vi "FGV_HovaCAL_Interface_Kommunikation.vi"(8 "error in":errorcluster, 9 "Logging":bool, 10 "Stop":bool, 11 "Aktion":T1) -> (0 "error out":errorcluster, 2 "connected?":bool, 3 "Aktion out":T1)   [LabVIEW 2020, in "Linearisierung v2.lvlib" / "Gasteiler.lvlib" / "HovaCAL_Interface.lvlib" / "Kommunikation.lvlib"]
uses:
  Kommunikation.lvlib
  Aktion_FGV_HovaCAL_Interface_Kommunikation.ctl
  Aktion_FGV_HovaCAL_Interface_GetData.ctl
  Aktion_FGV_HovaCAL_Interface_SetData.ctl
  Aktion_FGV_HovaCAL_Interface_Gasliste.ctl
  Aktionen FGV Gasteiler Daten.ctl
  KGN/KGN.lvlib
  Gasteiler.lvlib
  KGN/set/set.lvlib
  KGN/GUI Get/KGN GUI Get.lvlib
  KGN/GUI Set/KGN GUI Set.lvlib
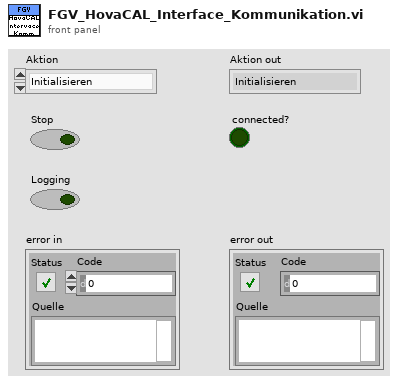
[diagram p1: front panel]
types:
  T1 = typedef "Linearisierung v2.lvlib/Gasteiler.lvlib/HovaCAL_Interface.lvlib/Kommunikation.lvlib/Aktion_FGV_HovaCAL_Interface_Kommunikation.ctl" = enum16{"Initialisieren", "Set Konzentrationen", "Set Gase", "Set Limits", "Get Dynamische Werte", "Beenden", "Com ändern", "Get Gase init", "Pause", "Get Gasteiler Infos", "Get MFC Infos", "Set Pumpen Parameter", "Set Pumpe Konzenration", "Set Pumpe run", "Set Temperaturen", "Set Fluss", "Get Gase", "Get Limits", "Get Dynamische Werte 1", "Get Dynamische Werte 2"}
  T2 = cluster{"first contact in":bool, "first actual values in ":bool}
  T3 = typedef "Linearisierung v2.lvlib/Gasteiler.lvlib/HovaCAL_Interface.lvlib/Kommunikation.lvlib/Aktion_FGV_HovaCAL_Interface_GetData.ctl" = enum16{"lesen", "SystemInfo", "MFC Info", "actual Values", "Limits", "first contact"}
  T4 = cluster{"Serial Settings:Baud Rate":u32, "Serial Settings:Data Bits":u16, "Serial Settings:Parity":u16, "Serial Settings:Stop Bits":u16, "Serial Settings:Flow Control":u16, "Enable Termination Char (T)":bool, "Message Based Settings:Termination Character":u8}
  T5 = typedef "Linearisierung v2.lvlib/Gasteiler.lvlib/HovaCAL_Interface.lvlib/Kommunikation.lvlib/Aktion_FGV_HovaCAL_Interface_SetData.ctl" = enum16{"lesen", "Konzentrationen", "Pumpen Parameter", "Pumpe Konzentration", "Pumpe run", "Temperaturen", "Fluss", "Limits", "init"}
  T6 = typedef "Linearisierung v2.lvlib/Gasteiler.lvlib/HovaCAL_Interface.lvlib/Kommunikation.lvlib/Aktion_FGV_HovaCAL_Interface_Gasliste.ctl" = enum16{"lesen", "setzen", "erstellen"}
  T7 = typedef "Linearisierung v2.lvlib/Gasteiler.lvlib/Aktionen FGV Gasteiler Daten.ctl" = enum16{"lesen", "Gasteiler Daten", "Seriellen Param.", "MB-Endwert", "laden", "speichern", "Anforderung", "TCP", "Aufzeichnung Start"}
  T8 = cluster{"input concentration setpoint":dbl, "output concentration setpoint":dbl}[]
  T9 = typedef "Linearisierung v2.lvlib/Gasteiler.lvlib/HovaCAL_Interface.lvlib/Controls.lvlib/Info Cluster.ctl" = cluster{"device":string, "version":string, "number of mfc":i32, "number of pumps":i32, "number of temp controllers":i32, "number of mfs":i32, "number of balances":i32}
  T10 = typedef "Linearisierung v2.lvlib/Gasteiler.lvlib/HovaCAL_Interface.lvlib/Controls.lvlib/Pump Concentration Mode.ctl" = i32
  T11 = typedef "Linearisierung v2.lvlib/Gasteiler.lvlib/HovaCAL_Interface.lvlib/Controls.lvlib/Reagent.ctl" = i32
  T12 = cluster{"concentratio mode":T10, "Reagent":T11, "Molarity":dbl, "density":dbl, "syringe":dbl, "pump_a":dbl}[]
  T13 = typedef "Linearisierung v2.lvlib/Gasteiler.lvlib/HovaCAL_Interface.lvlib/Controls.lvlib/Pump Concentration.ctl" = cluster{"reagent conc SP":dbl, "water conc SP":dbl}
  T14 = typedef "Linearisierung v2.lvlib/Gasteiler.lvlib/HovaCAL_Interface.lvlib/Controls.lvlib/Pump Dry Mode.ctl" = i32
  T15 = typedef "Linearisierung v2.lvlib/Gasteiler.lvlib/HovaCAL_Interface.lvlib/Controls.lvlib/Pump Control Mode.ctl" = u32
  T16 = cluster{"running?":bool, "dry mode":T14, "control mode":T15}
  T17 = cluster{"Input Concentrations (Ausgang)":cluster{"input concentration setpoint":dbl, "output concentration setpoint":dbl, "output concentration":dbl, "output concentration dry":dbl}[], "Cluster":cluster{"Temp Cluster":cluster{"temp SP":dbl, "temp":dbl, "humidity":dbl}[], "PumpModeGeneral-Cluster":cluster{"running?":bool, "dry mode":T14, "control mode":T15}, "PumpMode-Cluster":cluster{"Speed":dbl, "concentratio mode":T10, "Reagent":T11, "Molarity":dbl, "density":dbl, "syringe":dbl, "pumpe_a":dbl}[], "Pump Concentrations-Cluster":cluster{"reagent conc SP":dbl, "reagent conc":dbl, "reagent conc dry":dbl, "water conc SP":dbl, "water conc":dbl, "water conc dry":dbl}[], "Flow Output Cluster (Ausgang)":cluster{"total flow setpoint":dbl, "total flow":dbl}, "Pump MassFlow-Cluster":cluster{"reagent mf SP":dbl, "reagent mf":dbl, "water mf SP":dbl, "water mf":dbl, "water/reagent mf SP":dbl, "water/reagent mf":dbl}[], "MFC Flows-Cluster":cluster{"MFC  actual flow l/min":dbl, "MFC expected flow l/min":dbl}[]}}
  T18 = cluster{"Input Concentrations (Ausgang)":cluster{"input concentration setpoint":dbl, "output concentration setpoint":dbl, "output concentration":dbl, "output concentration dry":dbl}[], "Cluster":cluster{"Temp Cluster":cluster{"temp SP":dbl, "temp":dbl, "humidity":dbl}[], "PumpModeGeneral-Cluster":cluster{"running?":bool, "dry mode":T14, "control mode":T15}, "Flow Output Cluster (Ausgang)":cluster{"total flow setpoint":dbl, "total flow":dbl}, "MFC Flows (Ausgang)":cluster{"MFC  actual flow l/min":dbl, "MFC expected flow l/min":dbl}[]}}
  T19 = cluster{"input concentration setpoint":dbl, "output concentration setpoint":dbl, "output concentration":dbl, "output concentration dry":dbl}[]
  T20 = cluster{"temp SP":dbl, "temp":dbl, "humidity":dbl}[]
  T21 = cluster{"total flow setpoint":dbl, "total flow":dbl}
  T22 = cluster{"MFC  actual flow l/min":dbl, "MFC expected flow l/min":dbl}[]
  T23 = cluster{"Cluster":cluster{"PumpMode-Cluster":cluster{"Speed":dbl, "concentratio mode":T10, "Reagent":T11, "Molarity":dbl, "density":dbl, "syringe":dbl, "pumpe_a":dbl}[], "Pump Concentrations-Cluster":cluster{"reagent conc SP":dbl, "reagent conc":dbl, "reagent conc dry":dbl, "water conc SP":dbl, "water conc":dbl, "water conc dry":dbl}[], "Pump MassFlow-Cluster":cluster{"reagent mf SP":dbl, "reagent mf":dbl, "water mf SP":dbl, "water mf":dbl, "water/reagent mf SP":dbl, "water/reagent mf":dbl}[]}}
  T24 = cluster{"Speed":dbl, "concentratio mode":T10, "Reagent":T11, "Molarity":dbl, "density":dbl, "syringe":dbl, "pumpe_a":dbl}[]
  T25 = cluster{"reagent conc SP":dbl, "reagent conc":dbl, "reagent conc dry":dbl, "water conc SP":dbl, "water conc":dbl, "water conc dry":dbl}[]
  T26 = cluster{"reagent mf SP":dbl, "reagent mf":dbl, "water mf SP":dbl, "water mf":dbl, "water/reagent mf SP":dbl, "water/reagent mf":dbl}[]
  T27 = typedef "AK-Schnittstelle.lvlib/AK Seriell.lvlib/Serielle Parameter.ctl" = cluster{"VISA resource name":refnum<visa-resource-name>, "baud rate":u32, "data bits":u16, "parity":u16, "stop bits":u16, "flow control":u16}
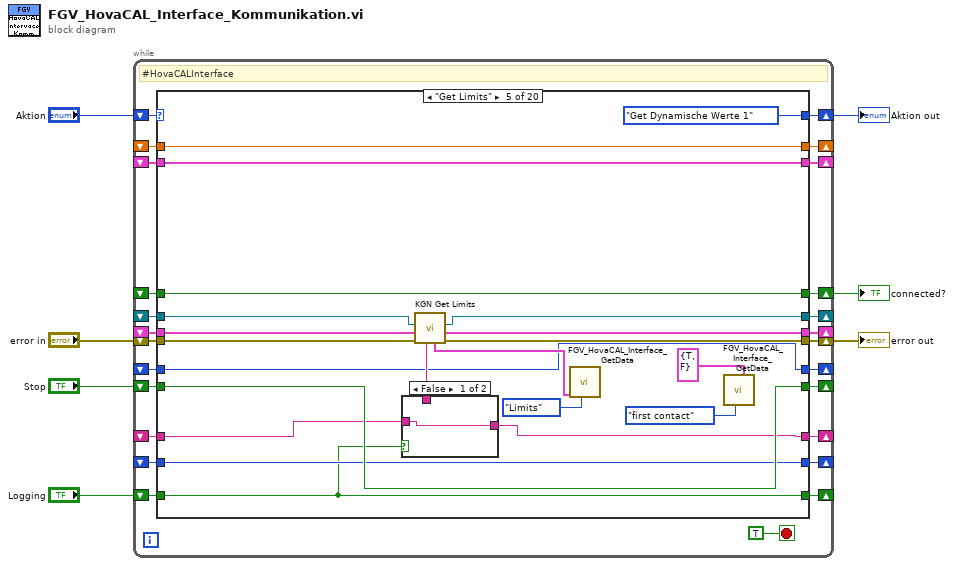
[diagram p0: block diagram]
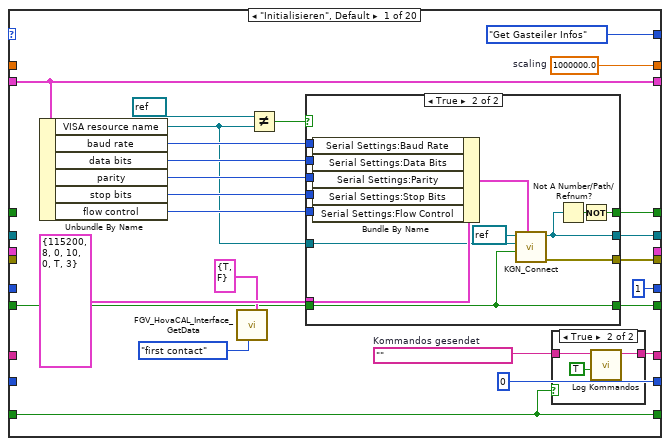
[diagram p2: hidden frame]
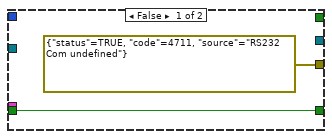
[diagram p4: hidden frame]
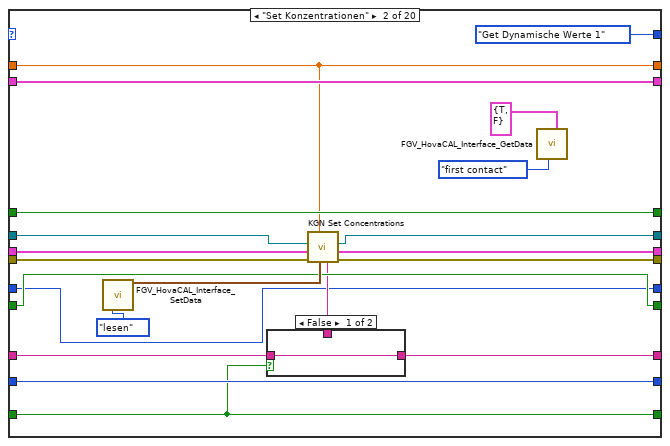
[diagram p5: hidden frame]
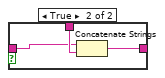
[diagram p6: hidden frame]
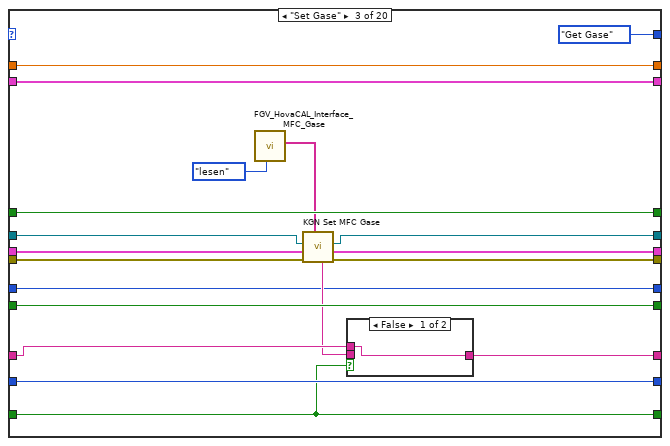
[diagram p7: hidden frame]
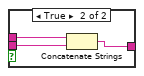
[diagram p8: hidden frame]
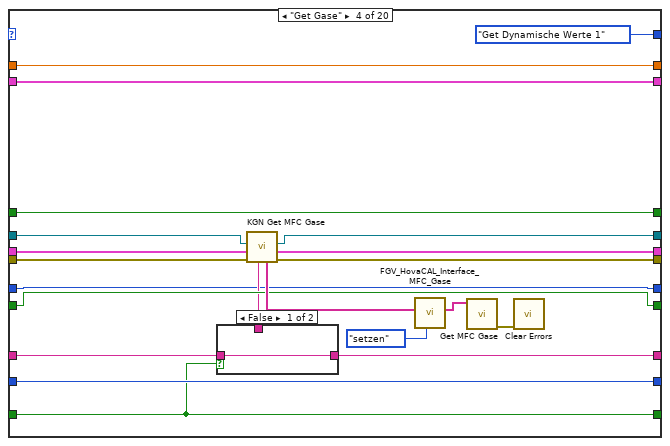
[diagram p9: hidden frame]
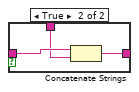
[diagram p10: hidden frame]
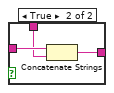
[diagram p11: hidden frame]
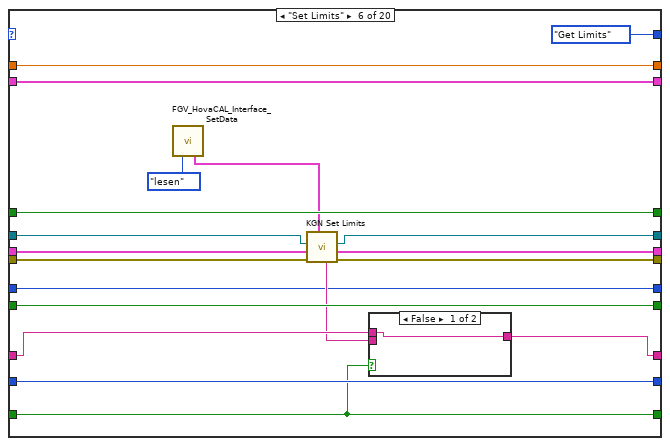
[diagram p12: hidden frame]
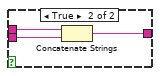
[diagram p13: hidden frame]
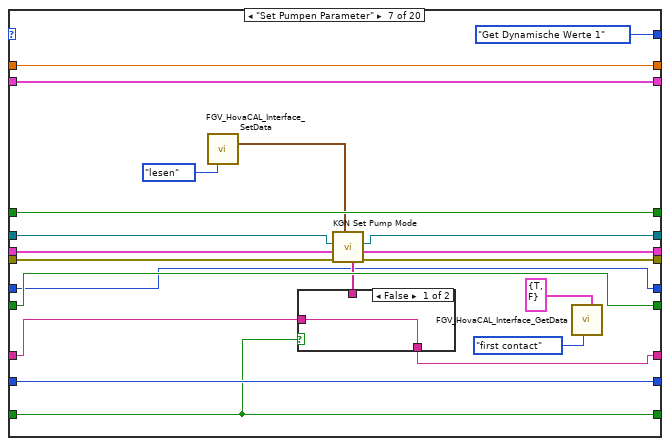
[diagram p14: hidden frame]
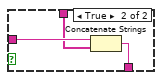
[diagram p15: hidden frame]
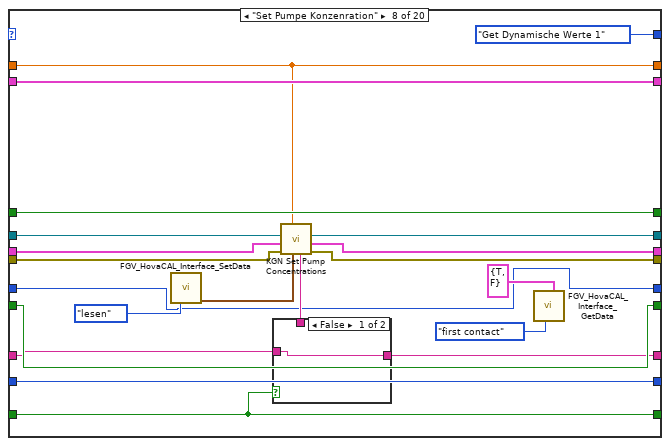
[diagram p16: hidden frame]
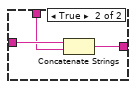
[diagram p17: hidden frame]
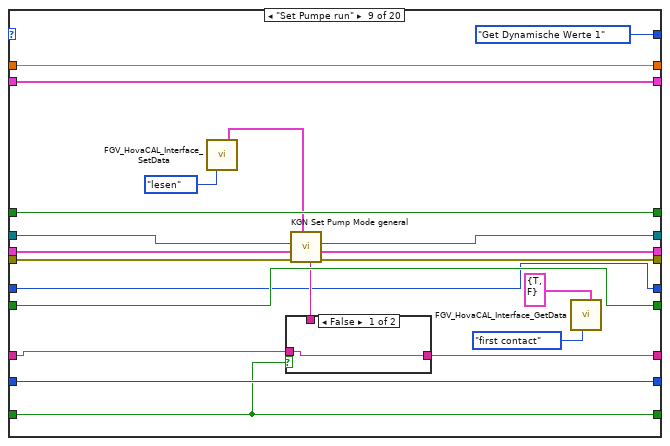
[diagram p18: hidden frame]
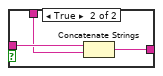
[diagram p19: hidden frame]
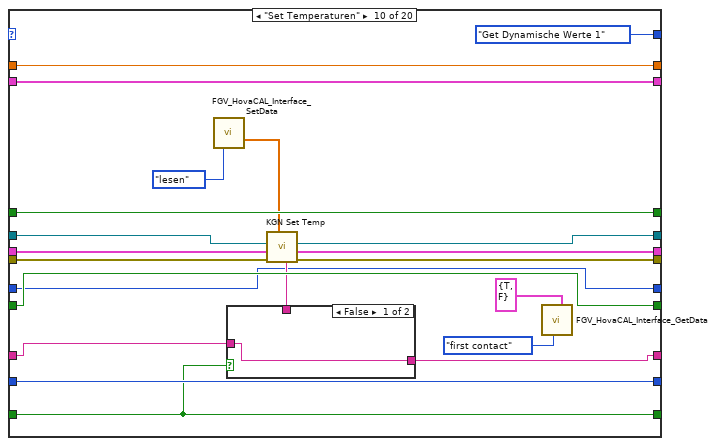
[diagram p20: hidden frame]
diagram:
  n1 = while {
    shift-right: [w29] -> w6
    shift-left: "error in" -> [w26]
    shift-right: [w31] -> _
    shift-left: _ -> [w30]
    shift-right: [w28] -> _
    shift-left: _ -> [w27]
    shift-right: [w25] -> w5
    shift-left: "Aktion" -> [w8]
    shift-right: [w24] -> _
    shift-left: _ -> [w23]
    shift-right: [w22] -> w4
    shift-left: _ -> [w21]
    shift-right: [w20] -> _
    shift-left: _ -> [w19]
    shift-right: [w17] -> _
    shift-left: "Stop" -> [w18]
    shift-right: [w16] -> _
    shift-left: _ -> [w15]
    shift-right: [w14] -> _
    shift-left: _ -> [w13]
    shift-right: [w11] -> _
    shift-left: "Logging" -> [w12]
    shift-right: [w10] -> _
    shift-left: _ -> [w9]
    stop <- TRUE stop-if-true
    # "#HovaCALInterface"
    n2 = case shown="\"Get Limits\"" w8 {
      selector: w8 -> [_ _ _ _ _ _ _ _ _ _ _ w334 w352 _ _ _ _ _ _ _]
      tunnel: [w56 w97 w120 w145 w170 w193 w218 w243 w268 w293 w317 w344 w380 w420 w453 w482 w492 w522 w548 w577] -> w31
      tunnel: w30 -> [w56 w97 w120 w145 w170 w193 w218 w243 w268 w293 w317 w344 w380 w420 w453 w482 w491 w522 w548 w577]
      tunnel: [w49 w90 w111 w136 w162 w184 w211 w236 w255 w287 w309 w340 w376 w416 w451 w479 w495 w514 w543 w563] -> w29
      tunnel: [w45 w94 w115 w140 w165 w188 w214 w238 w264 w285 w311 w342 w378 w418 w450 w481 w496 w517 w544 w565] -> w28
      tunnel: w27 -> [_ w95 w116 w141 w166 w189 w215 w241 w265 w289 w312 w343 w379 w419 w445 w481 w496 w518 w546 w575]
      tunnel: w26 -> [_ w91 w113 w138 w155 w187 w210 w237 w261 w288 w310 w341 w377 w417 w452 w479 w495 w513 w545 w574]
      tunnel: [Aktion_FGV_HovaCAL_Interface_Kommunikation."Get Gasteiler Infos" ("Aktion") Aktion_FGV_HovaCAL_Interface_Kommunikation."Get Dynamische Werte 1" ("Aktion") Aktion_FGV_HovaCAL_Interface_Kommunikation."Get Gase" ("Aktion") Aktion_FGV_HovaCAL_Interface_Kommunikation."Get Dynamische Werte 1" ("Aktion") Aktion_FGV_HovaCAL_Interface_Kommunikation."Get Dynamische Werte 1" ("Aktion") Aktion_FGV_HovaCAL_Interface_Kommunikation."Get Limits" ("Aktion") Aktion_FGV_HovaCAL_Interface_Kommunikation."Get Dynamische Werte 1" ("Aktion") Aktion_FGV_HovaCAL_Interface_Kommunikation."Get Dynamische Werte 1" ("Aktion") Aktion_FGV_HovaCAL_Interface_Kommunikation."Get Dynamische Werte 1" ("Aktion") Aktion_FGV_HovaCAL_Interface_Kommunikation."Get Dynamische Werte 1" ("Aktion") Aktion_FGV_HovaCAL_Interface_Kommunikation."Get Dynamische Werte 1" ("Aktion") w334 w351 Aktion_FGV_HovaCAL_Interface_Kommunikation."Get Dynamische Werte 1" ("Aktion") Aktion_FGV_HovaCAL_Interface_Kommunikation."Pause" ("Aktion") Aktion_FGV_HovaCAL_Interface_Kommunikation."Initialisieren" ("Aktion") w488 Aktion_FGV_HovaCAL_Interface_Kommunikation."Get Gase" ("Aktion") Aktion_FGV_HovaCAL_Interface_Kommunikation."Get MFC Infos" ("Aktion") Aktion_FGV_HovaCAL_Interface_Kommunikation."Get Gase init" ("Aktion")] -> w25
      tunnel: [_ w92 w112 w137 w163 w185 w212 w240 w262 w286 w316 w338 w374 w414 w448 w478 w494 w515 w540 w561] -> w24
      tunnel: w23 -> [_ w93 w114 w139 w164 w186 w213 w239 w263 w290 w316 w339 w375 w415 w448 w478 w494 w516 _ w572]
      tunnel: [w43 w96 w119 w144 w169 w192 w217 w242 w267 w292 w315 w335 w372 w412 w444 w477 w489 w520 w542 w573] -> w22
      tunnel: w21 -> [_ w96 w119 w144 w169 w192 w217 w242 w267 w292 w315 _ _ _ _ w477 w489 w520 w542 w573]
      tunnel: [w42 w89 w118 w143 w168 w191 w216 w235 w266 w291 w314 w333 w371 w411 w447 w476 w493 w519 w539 w569] -> w20
      tunnel: w19 -> [_ w89 w118 w143 w168 w191 w216 w235 w266 w291 w314 w333 w371 w411 w447 w476 w493 w519 w539 w569]
      tunnel: w18 -> [w39 w83 w108 w131 w157 w181 w204 w229 w254 w279 w304 w330 w359 w400 w441 w475 w487 w509 w535 w560]
      tunnel: [w38 w83 w108 w131 w157 w181 w204 w229 w254 w279 w304 w330 w359 w400 w441 w475 w487 w509 w535 w560] -> w17
      tunnel: [w35 w80 w105 w128 w154 w178 w202 w226 w251 w277 w301 w327 w356 w396 w437 w474 w486 w506 w531 w556] -> w16
      tunnel: w15 -> [_ w81 w107 w130 w156 w180 w203 w228 w253 w278 w303 w329 w357 w399 w440 w474 w486 w508 w530 w559]
      tunnel: [u32 0 w79 w104 w127 w152 w177 w200 w225 w250 w275 w300 w326 w354 w395 w438 w473 w485 w505 w529 w555] -> w14
      tunnel: w13 -> [_ w79 w104 w127 w152 w177 w200 w225 w250 w275 w300 w326 w354 w397 w438 w473 w485 w505 w529 w555]
      tunnel: w12 -> [w34 w78 w103 w126 w151 w176 w199 w224 w249 w274 w299 w325 w353 w394 w436 w472 w484 w504 w528 w554]
      tunnel: [w34 w78 w103 w126 w151 w176 w199 w224 w249 w274 w299 w325 w353 w394 w436 w472 w484 w504 w528 w554] -> w11
      tunnel: [u8 1 ("iteration out") w77 w102 w125 w150 w175 w198 w223 w248 w273 w298 w323 w349 w393 w435 w471 w483 w503 w527 w553] -> w10
      tunnel: w9 -> [_ w77 w102 w125 w150 w175 w198 w223 w248 w273 w298 w324 w350 w392 w435 w471 w483 w503 w527 w553]
      frame "Initialisieren", Default {
        w36 = ""  # Kommandos gesendet
        w42 = 1000000.0  # scaling
        n3 = Unbundle By Name(w56) -> ("VISA resource name"=w46:refnum<visa-resource-name>, "baud rate"=w54:u32, "data bits"=w53:u16, "parity"=w52:u16, "stop bits"=w51:u16, "flow control"=w50:u16)
        n4 = call "FGV_HovaCAL_Interface_GetData.vi"("first flags in"=T2 {"first contact in"=TRUE, "first actual values in "=FALSE}, "Aktion"=Aktion_FGV_HovaCAL_Interface_GetData."first contact") -> ()  [unwired: 5 in, 5 out]
        n5 = Not Equal?(x=refnum<visa-resource-name> refnum ("VISA-Ressourcenname"), y=w46) -> (x != y?=w47:bool)
        n6 = case shown="True" w47 {
          tunnel: T4 {"Serial Settings:Baud Rate"=115200, "Serial Settings:Data Bits"=8, "Serial Settings:Parity"=0, "Serial Settings:Stop Bits"=10, "Serial Settings:Flow Control"=0, "Enable Termination Char (T)"=TRUE, "Message Based Settings:Termination Character"=3} ("Serial Params in") -> [_ w76]
          tunnel: w54 -> [_ w74]
          tunnel: w53 -> [_ w73]
          tunnel: w52 -> [_ w72]
          tunnel: w51 -> [_ w71]
          tunnel: w50 -> [_ w70]
          tunnel: [errorcluster {"status"=TRUE, "code"=4711, "source"="RS232 Com undefined"} ("Fehler (Ausgang)") w69] -> w49
          tunnel: w46 -> [_ w68]
          tunnel: [_ w65] -> w45
          tunnel: [_ w64] -> w43
          tunnel: w39 -> [w61 w63]
          tunnel: [w61 w63] -> w38
          frame False {
          }
          frame True {
            n7 = Bundle By Name(cluster=w76, "Serial Settings:Baud Rate"=w74, "Serial Settings:Data Bits"=w73, "Serial Settings:Parity"=w72, "Serial Settings:Stop Bits"=w71, "Serial Settings:Flow Control"=w70) -> (w75:T4)
            n8 = call "KGN_Connect.vi"("Serial Params in"=w75, "Stopp"=w63, "serial port name"=w68, "VISA-Ressourcenname"=refnum<visa-resource-name> refnum) -> ("Fehler (Ausgang)"=w69:errorcluster, "VISA-Ressourcenname (Ausgang)"=w65:refnum<visa-resource-name>)  [unwired: 4 in, 2 out]
            n9 = Not A Number/Path/Refnum?(number/path/refnum=w65) -> (NaN/Path/Refnum?=w66:bool)
            n10 = Not(x=w66) -> (.not. x?=w64:bool)
          }
        }
        n11 = case shown="True" w34 {
          tunnel: w36 -> [w57 w60]
          tunnel: [w57 w59] -> w35
          frame False {
          }
          frame True {
            n12 = call "Log Kommandos.vi"("Init"=TRUE, "Kommandos"=w60) -> ("Kommandos out"=w59:string)  [unwired: 9 in]
          }
        }
      }
      frame "Set Konzentrationen" {
        n13 = call "FGV_HovaCAL_Interface_SetData.vi"("Aktion"=Aktion_FGV_HovaCAL_Interface_SetData."lesen") -> ("Set Values Cluster out"=w86:T8)  [unwired: 8 in, 6 out]
        n14 = call "KGN Set Concentrations.vi"("Set Values Cluster"=w86, "scaling"=w89, "Fehler (Eingang, kein Fehler)"=w91, "Info Cluster"=w93, "VISA-Referenz (Eingang)"=w95) -> ("Fehler (Ausgang)"=w90:errorcluster, "Info Cluster out"=w92:T9, "VISA-Referenz (Ausgang)"=w94:refnum<visa-resource-name>, "Kommandos gesendet"=w82:string)  [unwired: 2 in, 1 out]
        n15 = case shown="False" w78 {
          tunnel: w82 -> [_ w101]
          tunnel: w81 -> [w98 w100]
          tunnel: [w98 w99] -> w80
          frame False {
          }
          frame True {
            n16 = Concatenate Strings(w100, w101) -> (w99:string)
          }
        }
        n17 = call "FGV_HovaCAL_Interface_GetData.vi"("first flags in"=T2 {"first contact in"=TRUE, "first actual values in "=FALSE}, "Aktion"=Aktion_FGV_HovaCAL_Interface_GetData."first contact") -> ()  [unwired: 5 in, 5 out]
      }
      frame "Set Gase" {
        n18 = call "FGV_HovaCAL_Interface_MFC_Gase.vi"("Aktion"=Aktion_FGV_HovaCAL_Interface_Gasliste."lesen") -> ("mfc Gasnamen out"=w109:string[])  [unwired: 8 in, 2 out]
        n19 = call "KGN Set MFC Gase.vi"("mfc Gasnamen in"=w109, "Fehler (Eingang, kein Fehler)"=w113, "Info Cluster"=w114, "VISA-Referenz (Eingang)"=w116) -> ("Fehler (Ausgang)"=w111:errorcluster, "Info Cluster out"=w112:T9, "VISA-Referenz (Ausgang)"=w115:refnum<visa-resource-name>, "Kommandos gesendet"=w106:string)  [unwired: 3 in, 1 out]
        n20 = case shown="False" w103 {
          tunnel: w107 -> [w121 w124]
          tunnel: w106 -> [_ w123]
          tunnel: [w121 w122] -> w105
          frame False {
          }
          frame True {
            n21 = Concatenate Strings(w124, w123) -> (w122:string)
          }
        }
      }
      frame "Get Gase" {
        n22 = call "KGN Get MFC Gase.vi"("Fehler (Eingang, kein Fehler)"=w138, "Info Cluster"=w139, "VISA-Ressourcenname"=w141) -> ("Fehler (Ausgang)"=w136:errorcluster, "Info Cluster out"=w137:T9, "VISA-Ressourcenname out"=w140:refnum<visa-resource-name>, "mfc Gas"=w134:string[], "Kommandos gesendet"=w129:string)  [unwired: 3 in, 1 out]
        n23 = case shown="False" w126 {
          tunnel: w130 -> [w146 w149]
          tunnel: w129 -> [_ w148]
          tunnel: [w146 w147] -> w128
          frame False {
          }
          frame True {
            n24 = Concatenate Strings(w149, w148) -> (w147:string)
          }
        }
        n25 = call "FGV_HovaCAL_Interface_MFC_Gase.vi"("Aktion"=Aktion_FGV_HovaCAL_Interface_Gasliste."setzen", "mfc Gasnamen in"=w134) -> ("mfc Gasnamen out"=w133:string[])  [unwired: 7 in, 2 out]
        n26 = call "Get MFC Gase.vi"("mfc Gasnamen in"=w133) -> ("Fehler (Ausgang)"=w132:errorcluster)  [unwired: 10 in]
        n27 = call <vilib>:"Clear Errors.vi"("error in (no error)"=w132) -> ()  [unwired: 5 in, 2 out]
      }
      frame "Get Limits" {
        n28 = call "KGN Get Limits.vi"("Fehler (Eingang, kein Fehler)"=w155, "Info Cluster"=w164, "VISA-Ressourcenname"=w166) -> ("Fehler (Ausgang)"=w162:errorcluster, "Info Cluster out"=w163:T9, "VISA-Ressourcenname out"=w165:refnum<visa-resource-name>, "Limits Cluster out"=w160:cluster{"flow":dbl[], "temp":dbl[]}, "Kommnados gesendet"=w153:string)  [unwired: 3 in, 1 out]
        n29 = case shown="False" w151 {
          tunnel: w156 -> [w171 w174]
          tunnel: [w171 w173] -> w154
          tunnel: w153 -> [_ w172]
          frame False {
          }
          frame True {
            n30 = Concatenate Strings(w174, w172) -> (w173:string)
          }
        }
        n31 = call "FGV_HovaCAL_Interface_GetData.vi"("Aktion"=Aktion_FGV_HovaCAL_Interface_GetData."Limits", "Limits Cluster in"=w160) -> ()  [unwired: 5 in, 5 out]
        n32 = call "FGV_HovaCAL_Interface_GetData.vi"("first flags in"=T2 {"first contact in"=TRUE, "first actual values in "=FALSE}, "Aktion"=Aktion_FGV_HovaCAL_Interface_GetData."first contact") -> ()  [unwired: 5 in, 5 out]
      }
      frame "Set Limits" {
        n33 = call "FGV_HovaCAL_Interface_SetData.vi"("Aktion"=Aktion_FGV_HovaCAL_Interface_SetData."lesen") -> ("Limits Cluster out"=w182:cluster{"flow":dbl[], "temp":dbl[]})  [unwired: 8 in, 6 out]
        n34 = call "KGN Set Limits.vi"("Limits Cluster in"=w182, "Fehler (Eingang, kein Fehler)"=w187, "Info Cluster"=w186, "VISA-Referenz (Eingang)"=w189) -> ("Fehler (Ausgang)"=w184:errorcluster, "Info Cluster out"=w185:T9, "VISA-Referenz (Ausgang)"=w188:refnum<visa-resource-name>, "Kommandos gesendet"=w179:string)  [unwired: 3 in, 1 out]
        n35 = case shown="False" w176 {
          tunnel: w180 -> [w194 w197]
          tunnel: w179 -> [_ w196]
          tunnel: [w194 w195] -> w178
          frame False {
          }
          frame True {
            n36 = Concatenate Strings(w197, w196) -> (w195:string)
          }
        }
      }
      frame "Set Pumpen Parameter" {
        n37 = call "FGV_HovaCAL_Interface_SetData.vi"("Aktion"=Aktion_FGV_HovaCAL_Interface_SetData."lesen") -> ("PumpMode-Cluster out"=w208:T12)  [unwired: 8 in, 6 out]
        n38 = call "KGN Set Pump Mode.vi"("PumpMode-Cluster"=w208, "Fehler (Eingang, kein Fehler)"=w210, "Info Cluster"=w213, "VISA-Referenz (Eingang)"=w215) -> ("Fehler (Ausgang)"=w211:errorcluster, "Info Cluster out"=w212:T9, "VISA-Referenz (Ausgang)"=w214:refnum<visa-resource-name>, "Kommandos gesendet"=w201:string[])  [unwired: 3 in, 1 out]
        n39 = case shown="False" w199 {
          tunnel: w203 -> [w219 w222]
          tunnel: [w219 w221] -> w202
          tunnel: w201 -> [_ w220]
          frame False {
          }
          frame True {
            n40 = Concatenate Strings(w222, w220) -> (w221:string)
          }
        }
        n41 = call "FGV_HovaCAL_Interface_GetData.vi"("first flags in"=T2 {"first contact in"=TRUE, "first actual values in "=FALSE}, "Aktion"=Aktion_FGV_HovaCAL_Interface_GetData."first contact") -> ()  [unwired: 5 in, 5 out]
      }
      frame "Set Pumpe Konzenration" {
        n42 = call "FGV_HovaCAL_Interface_SetData.vi"("Aktion"=Aktion_FGV_HovaCAL_Interface_SetData."lesen") -> ("Pump Concentrations-Cluster out"=w232:T13[])  [unwired: 8 in, 6 out]
        n43 = call "KGN Set Pump Concentrations.vi"("Pump Concentrations-Cluster"=w232, "scaling"=w235, "Fehler (Eingang, kein Fehler)"=w237, "Info Cluster"=w239, "VISA-Referenz (Eingang)"=w241) -> ("Fehler (Ausgang)"=w236:errorcluster, "Info Cluster out"=w240:T9, "VISA-Referenz (Ausgang)"=w238:refnum<visa-resource-name>, "Kommandos gesendet"=w227:string)  [unwired: 2 in, 1 out]
        n44 = case shown="False" w224 {
          tunnel: w228 -> [w244 w247]
          tunnel: w227 -> [_ w246]
          tunnel: [w244 w245] -> w226
          frame False {
          }
          frame True {
            n45 = Concatenate Strings(w247, w246) -> (w245:string)
          }
        }
        n46 = call "FGV_HovaCAL_Interface_GetData.vi"("first flags in"=T2 {"first contact in"=TRUE, "first actual values in "=FALSE}, "Aktion"=Aktion_FGV_HovaCAL_Interface_GetData."first contact") -> ()  [unwired: 5 in, 5 out]
      }
      frame "Set Pumpe run" {
        n47 = call "FGV_HovaCAL_Interface_SetData.vi"("Aktion"=Aktion_FGV_HovaCAL_Interface_SetData."lesen") -> ("PumpModeGeneral-Cluster out"=w258:T16)  [unwired: 8 in, 6 out]
        n48 = call "KGN Set Pump Mode general.vi"("PumpModeGeneral-Cluster"=w258, "Fehler (Eingang, kein Fehler)"=w261, "Info Cluster"=w263, "VISA-Referenz (Eingang)"=w265) -> ("Fehler (Ausgang)"=w255:errorcluster, "Info Cluster out"=w262:T9, "VISA-Referenz (Ausgang)"=w264:refnum<visa-resource-name>, "Kommandos gesendet"=w252:string)  [unwired: 3 in, 1 out]
        n49 = case shown="False" w249 {
          tunnel: w253 -> [w269 w272]
          tunnel: w252 -> [_ w271]
          tunnel: [w269 w270] -> w251
          frame False {
          }
          frame True {
            n50 = Concatenate Strings(w272, w271) -> (w270:string)
          }
        }
        n51 = call "FGV_HovaCAL_Interface_GetData.vi"("first flags in"=T2 {"first contact in"=TRUE, "first actual values in "=FALSE}, "Aktion"=Aktion_FGV_HovaCAL_Interface_GetData."first contact") -> ()  [unwired: 5 in, 5 out]
      }
      frame "Set Temperaturen" {
        n52 = call "FGV_HovaCAL_Interface_SetData.vi"("Aktion"=Aktion_FGV_HovaCAL_Interface_SetData."lesen") -> ("Temperature out"=w283:dbl[])  [unwired: 8 in, 6 out]
        n53 = call "KGN Set Temp.vi"("Temperature"=w283, "Fehler (Eingang, kein Fehler)"=w288, "Info Cluster"=w290, "VISA-Referenz (Eingang)"=w289) -> ("Fehler (Ausgang)"=w287:errorcluster, "Info Cluster out"=w286:T9, "VISA-Referenz (Ausgang)"=w285:refnum<visa-resource-name>, "Kommandos gesendet"=w276:string)  [unwired: 3 in, 1 out]
        n54 = case shown="False" w274 {
          tunnel: w278 -> [w294 w297]
          tunnel: [w294 w296] -> w277
          tunnel: w276 -> [_ w295]
          frame False {
          }
          frame True {
            n55 = Concatenate Strings(w297, w295) -> (w296:string)
          }
        }
        n56 = call "FGV_HovaCAL_Interface_GetData.vi"("first flags in"=T2 {"first contact in"=TRUE, "first actual values in "=FALSE}, "Aktion"=Aktion_FGV_HovaCAL_Interface_GetData."first contact") -> ()  [unwired: 5 in, 5 out]
      }
      frame "Set Fluss" {
        n57 = call "FGV_HovaCAL_Interface_SetData.vi"("Aktion"=Aktion_FGV_HovaCAL_Interface_SetData."lesen") -> ("total flow setpoint out"=w307:dbl)  [unwired: 8 in, 6 out]
        n58 = call "KG set total flow sp.vi"("Fehler (Eingang, kein Fehler)"=w310, "total flow setpoint"=w307, "VISA-Ressourcenname"=w312) -> ("Fehler (Ausgang)"=w309:errorcluster, "Kommando gesendet"=w302:string, "VISA-Ressourcenname (Ausgang)"=w311:refnum<visa-resource-name>)  [unwired: 6 in]
        n59 = case shown="True" w299 {
          tunnel: w303 -> [w318 w322]
          tunnel: w302 -> [_ w321]
          tunnel: [w318 w319] -> w301
          frame False {
          }
          frame True {
            n60 = Concatenate Strings(w322, w321, "\r\n") -> (w319:string)
          }
        }
        n61 = call "FGV_HovaCAL_Interface_GetData.vi"("first flags in"=T2 {"first contact in"=TRUE, "first actual values in "=FALSE}, "Aktion"=Aktion_FGV_HovaCAL_Interface_GetData."first contact") -> ()  [unwired: 5 in, 5 out]
      }
      frame "Get Dynamische Werte" {
        n62 = call "KGN Get actual Values.vi"("scaling"=w333, "Fehler (Eingang, kein Fehler)"=w341, "Info Cluster"=w339, "VISA-Referenz (Eingang)"=w343) -> ("Fehler (Ausgang)"=w340:errorcluster, "Info Cluster out"=w338:T9, "VISA-Referenz (Ausgang)"=w342:refnum<visa-resource-name>, "actual Values Cluster"=w336:T17, "Kommandos gesendet"=w328:string, "connected"=w335:bool)  [unwired: 1 in, 1 out]
        n63 = call "FGV_HovaCAL_Interface_GetData.vi"("Aktion"=Aktion_FGV_HovaCAL_Interface_GetData."actual Values", "actual Values Cluster in"=w336) -> ("Limits Cluster out"=w331:cluster{"flow":dbl[], "temp":dbl[]}, "first flags out"=w332:T2)  [unwired: 5 in, 3 out]
        n64 = call "Set FirstContactFlags.vi"("Limits Cluster in"=w331, "iteration in"=w324, "first flags in"=w332) -> ("iteration out"=w323:u8)  [unwired: 7 in, 1 out]
        n65 = case shown="False" w325 {
          tunnel: w329 -> [w345 w348]
          tunnel: w328 -> [_ w347]
          tunnel: [w345 w346] -> w327
          frame False {
          }
          frame True {
            n66 = Concatenate Strings(w348, w347) -> (w346:string)
          }
        }
      }
      frame "Get Dynamische Werte 1" {
        n67 = call "FGV_HovaCAL_Interface_GetData.vi"("Aktion"=Aktion_FGV_HovaCAL_Interface_GetData."lesen") -> ("actual Values Cluster out"=w369:T17, "first flags out"=w362:T2)  [unwired: 6 in, 3 out]
        n68 = call "KGN Get actual Values 1.vi"("scaling"=w371, "Fehler (Eingang, kein Fehler)"=w377, "Info Cluster"=w375, "VISA-Referenz (Eingang)"=w379) -> ("Fehler (Ausgang)"=w376:errorcluster, "Info Cluster out"=w374:T9, "VISA-Referenz (Ausgang)"=w378:refnum<visa-resource-name>, "actual Values Cluster"=w363:T18, "Kommandos gesendet"=w355:string, "connected"=w372:bool)  [unwired: 1 in, 1 out]
        n69 = Unbundle By Name(w363) -> ()  [unwired: 1 out]
        n70 = Unbundle By Name(w363) -> ("Input Concentrations (Ausgang)"=w367:T19, "Cluster.Temp Cluster"=w366:T20, "Cluster.PumpModeGeneral-Cluster"=w365:T16, "Cluster.Flow Output Cluster (Ausgang)"=w364:T21, "Cluster.MFC Flows (Ausgang)"=w358:T22)
        n71 = case shown="True" w353 {
          tunnel: w357 -> [w381 w384]
          tunnel: [w381 w383] -> w356
          tunnel: w355 -> [_ w382]
          frame False {
          }
          frame True {
            n72 = Concatenate Strings(w384, w382) -> (w383:string)
          }
        }
        n73 = Bundle By Name(cluster=w369, "Input Concentrations (Ausgang)"=w367, "Cluster.Temp Cluster"=w366, "Cluster.PumpModeGeneral-Cluster"=w365, "Cluster.Flow Output Cluster (Ausgang)"=w364, "Cluster.MFC Flows-Cluster"=w358) -> (w368:T17)
        n74 = call "FGV_HovaCAL_Interface_GetData.vi"("Aktion"=Aktion_FGV_HovaCAL_Interface_GetData."actual Values", "actual Values Cluster in"=w368) -> ("Limits Cluster out"=w361:cluster{"flow":dbl[], "temp":dbl[]})  [unwired: 5 in, 4 out]
        n75 = case shown="True" TRUE {
          tunnel: w352 -> [w387 _]
          tunnel: [w387 Aktion_FGV_HovaCAL_Interface_Kommunikation."Get Dynamische Werte 2" ("f")] -> w351
          tunnel: w362 -> [w389 _]
          tunnel: w361 -> [w388 _]
          tunnel: w350 -> [w386 w390]
          tunnel: [w385 w390] -> w349
          frame False {
            n76 = call "Set FirstContactFlags.vi"("Limits Cluster in"=w388, "iteration in"=w386, "first flags in"=w389) -> ("iteration out"=w385:u8)  [unwired: 7 in, 1 out]
          }
          frame True {
            # "immer, sonst werden Pumpenparameter auch <\nüberschreiben ..."
          }
        }
      }
      frame "Get Dynamische Werte 2" {
        n77 = call "FGV_HovaCAL_Interface_GetData.vi"("Aktion"=Aktion_FGV_HovaCAL_Interface_GetData."lesen") -> ("actual Values Cluster out"=w408:T17, "first flags out"=w402:T2)  [unwired: 6 in, 3 out]
        n78 = call "KGN Get actual Values 2.vi"("scaling"=w411, "Fehler (Eingang, kein Fehler)"=w417, "Info Cluster"=w415, "VISA-Referenz (Eingang)"=w419) -> ("Fehler (Ausgang)"=w416:errorcluster, "Info Cluster out"=w414:T9, "VISA-Referenz (Ausgang)"=w418:refnum<visa-resource-name>, "actual Values Cluster"=w409:T23, "Kommandos gesendet"=w398:string, "connected"=w412:bool)  [unwired: 1 in, 1 out]
        n79 = Unbundle By Name(w409) -> ("Cluster.PumpMode-Cluster"=w406:T24, "Cluster.Pump Concentrations-Cluster"=w405:T25, "Cluster.Pump MassFlow-Cluster"=w404:T26)
        n80 = case shown="True" w394 {
          tunnel: w399 -> [w422 w431]
          tunnel: w398 -> [_ w430]
          tunnel: w397 -> [w421 w429]
          tunnel: [w422 w425] -> w396
          tunnel: [w421 w423] -> w395
          frame False {
          }
          frame True {
            n81 = Increment(x=w429) -> (x+1=w424:u32)
            n82 = Concatenate Strings(w431, w430) -> (w426:string)
            n83 = Greater?(x=w424, y=u32 50) -> (0:w427:bool)
            n84 = case shown="True" w427 {
              tunnel: w426 -> [w433 w434]
              tunnel: [w433 _] -> w425
              tunnel: w424 -> [w432 _]
              tunnel: [w432 _] -> w423
              frame False {
              }
              frame True {
                n85 = call "Log Kommandos.vi"("Kommandos"=w434) -> ()  [unwired: 10 in, 1 out]
              }
            }
          }
        }
        n86 = Bundle By Name(cluster=w408, "Cluster.PumpMode-Cluster"=w406, "Cluster.Pump Concentrations-Cluster"=w405, "Cluster.Pump MassFlow-Cluster"=w404) -> (w407:T17)
        n87 = call "FGV_HovaCAL_Interface_GetData.vi"("Aktion"=Aktion_FGV_HovaCAL_Interface_GetData."actual Values", "actual Values Cluster in"=w407) -> ("Limits Cluster out"=w401:cluster{"flow":dbl[], "temp":dbl[]})  [unwired: 5 in, 4 out]
        n88 = call "Set FirstContactFlags.vi"("Limits Cluster in"=w401, "iteration in"=w392, "first flags in"=w402) -> ("iteration out"=w393:u8)  [unwired: 7 in, 1 out]
      }
      frame "Beenden" {
        n89 = Not A Number/Path/Refnum?(number/path/refnum=w445) -> (NaN/Path/Refnum?=w446:bool)
        n90 = Not(x=w446) -> (.not. x?=w444:bool)
        n91 = case shown="True" w444 {
          tunnel: w445 -> [w459 w467]
          tunnel: w452 -> [_ w466]
          tunnel: [_ w465] -> w451
          tunnel: [w459 w464] -> w450
          tunnel: [_ w460] -> w439
          frame False {
          }
          frame True {
            w461 = "\r\n"
            n92 = call "KG set run.vi"("Fehler (Eingang, kein Fehler)"=w466, "run"=FALSE, "VISA-Ressourcenname"=w467) -> ("Fehler (Ausgang)"=w468:errorcluster, "Kommando gesendet"=w463:string, "VISA-Ressourcenname (Ausgang)"=w469:refnum<visa-resource-name>)  [unwired: 6 in]
            n93 = call "KGN beenden.vi"("Fehler (Eingang, kein Fehler)"=w468, "VISA-Ressourcenname"=w469) -> ("Fehler (Ausgang)"=w465:errorcluster, "Kommandos gesendet"=w462:string, "VISA-Ressourcenname (Ausgang)"=w464:refnum<visa-resource-name>)  [unwired: 7 in]
            n94 = Concatenate Strings(w463, w461, w462, w461) -> (w460:string)
          }
        }
        n95 = case shown="False" w436 {
          tunnel: w440 -> [w454 w458]
          tunnel: w439 -> [_ w457]
          tunnel: [w454 w455] -> w437
          frame False {
          }
          frame True {
            n96 = Concatenate Strings(w458, w457) -> (w456:string)
            n97 = call "Log Kommandos.vi"("Kommandos"=w456) -> ("Kommandos out"=w455:string)  [unwired: 10 in]
          }
        }
        n98 = call "FGV_HovaCAL_Interface_GetData.vi"("first flags in"=T2 {"first contact in"=FALSE, "first actual values in "=FALSE}, "Aktion"=Aktion_FGV_HovaCAL_Interface_GetData."first contact") -> ()  [unwired: 5 in, 5 out]
      }
      frame "Pause" {
      }
      frame "Com ändern" {
        # "Beim ersten Aufruf der LinV2 wird die Com gesetzt,\ndamit sie erstmalig vorbelegt ist ... könnte man auch beim Laden der Gasteiler Konfig machen?\nJedenfalls wird das dann jedesmal beim Bildwechsel gemacht, muss also dann ignoriert werden.\nSonst könnte man gleich hier das Beenden rein hauen ... \nOder hier vergeleichen, ob anders ... !"
        n99 = call "FGV Gasteiler.vi"("Aktionen"=Aktionen_FGV_Gasteiler_Daten."lesen") -> ("Serielle Parameter"=w492:T27)  [unwired: 11 in, 7 out]
        n100 = Not Equal?(x=w492, y=w491) -> (x != y?=w490:bool)
        n101 = case shown="False" w490 {
          tunnel: w489 -> [w499 _]
          tunnel: [w498 Aktion_FGV_HovaCAL_Interface_Kommunikation."Beenden" ("Aktion")] -> w488
          frame False {
            n102 = case shown="False" w499 {
              tunnel: [Aktion_FGV_HovaCAL_Interface_Kommunikation."Initialisieren" ("Aktion") Aktion_FGV_HovaCAL_Interface_Kommunikation."Get Dynamische Werte 1" ("Aktion")] -> w498
              frame False {
              }
              frame True {
              }
            }
          }
          frame True {
          }
        }
      }
      frame "Get Gase init" {
        n103 = call "KGN Get MFC Gaslist.vi"("Fehler (Eingang, kein Fehler)"=w513, "Info Cluster"=w516, "VISA-Ressourcenname"=w518) -> ("Fehler (Ausgang)"=w514:errorcluster, "Info Cluster out"=w515:T9, "VISA-Ressourcenname out"=w517:refnum<visa-resource-name>, "mfc Gasnamen"=w512:string[][], "Kommandos gesendet"=w507:string)  [unwired: 3 in, 1 out]
        n104 = case shown="False" w504 {
          tunnel: w508 -> [w523 w526]
          tunnel: w507 -> [_ w525]
          tunnel: [w523 w524] -> w506
          frame False {
          }
          frame True {
            n105 = Concatenate Strings(w526, w525) -> (w524:string)
          }
        }
        n106 = call "FGV_HovaCAL_Interface_MFC_Gase.vi"("Aktion"=Aktion_FGV_HovaCAL_Interface_Gasliste."erstellen", "mfc Gaslisten in"=w512) -> ("mfc Gaslisten out"=w510:string[][])  [unwired: 7 in, 2 out]
        n107 = call "Init MFC Gaslisten.vi"("mfc Gaslisten in"=w510) -> ()  [unwired: 10 in, 1 out]
      }
      frame "Get Gasteiler Infos" {
        n108 = call "KGN Get Info.vi"("Fehler (Eingang, kein Fehler)"=w545, "VISA-Ressourcenname"=w546) -> ("Fehler (Ausgang)"=w543:errorcluster, "System Cluster"=w540:T9, "VISA-Ressourcenname out"=w544:refnum<visa-resource-name>, "Kommandos gesendet"=w532:string)  [unwired: 5 in, 1 out]
        n109 = case shown="True" w528 {
          tunnel: w532 -> [_ w552]
          tunnel: [w549 w551] -> w531
          tunnel: w530 -> [w549 w550]
          frame False {
          }
          frame True {
            n110 = Concatenate Strings(w550, w552) -> (w551:string)
          }
        }
        n111 = call "FGV_HovaCAL_Interface_GetData.vi"("Aktion"=Aktion_FGV_HovaCAL_Interface_GetData."SystemInfo", "System Cluster in"=w540) -> ("System Cluster out"=w534:T9)  [unwired: 5 in, 4 out]
        n112 = call "FGV_HovaCAL_Interface_SetData.vi"("System Cluster in"=w534, "Aktion"=Aktion_FGV_HovaCAL_Interface_SetData."init") -> ()  [unwired: 7 in, 7 out]
        n113 = call "Init_Controls.vi"("Info Cluster"=w534) -> ("Fehler (Ausgang)"=w537:errorcluster, "first flags out"=w536:T2)  [unwired: 9 in]
        n114 = call <vilib>:"Clear Errors.vi"("error in (no error)"=w537) -> ()  [unwired: 5 in, 2 out]
        n115 = call "FGV_HovaCAL_Interface_GetData.vi"("first flags in"=w536, "Aktion"=Aktion_FGV_HovaCAL_Interface_GetData."first contact") -> ()  [unwired: 5 in, 5 out]
      }
      frame "Get MFC Infos" {
        n116 = call "KGN Get MFC Flows.vi"("Fehler (Eingang, kein Fehler)"=w574, "Info Cluster"=w572, "VISA-Ressourcenname"=w575) -> ("Fehler (Ausgang)"=w564:errorcluster, "Info Cluster out"=w562:T9, "VISA-Ressourcenname out"=w566:refnum<visa-resource-name>, "MFC Flow Cluster"=w570:cluster{"min flow":dbl, "max flow":dbl}[], "Kommandos gesendet"=w558:string)  [unwired: 3 in, 1 out]
        n117 = call "FGV_HovaCAL_Interface_GetData.vi"("Aktion"=Aktion_FGV_HovaCAL_Interface_GetData."MFC Info", "MFC Flow Cluster in"=w570) -> ()  [unwired: 5 in, 5 out]
        n118 = call "KGN Get Limits.vi"("Fehler (Eingang, kein Fehler)"=w564, "Info Cluster"=w562, "VISA-Ressourcenname"=w566) -> ("Fehler (Ausgang)"=w563:errorcluster, "Info Cluster out"=w561:T9, "VISA-Ressourcenname out"=w565:refnum<visa-resource-name>, "Limits Cluster out"=w567:cluster{"flow":dbl[], "temp":dbl[]}, "Kommnados gesendet"=w557:string)  [unwired: 3 in, 1 out]
        n119 = case shown="False" w554 {
          tunnel: w559 -> [w578 w583]
          tunnel: w558 -> [_ w582]
          tunnel: w557 -> [_ w580]
          tunnel: [w578 w579] -> w556
          frame False {
          }
          frame True {
            n120 = Concatenate Strings(w583, w582) -> (w581:string)
            n121 = Concatenate Strings(w581, w580) -> (w579:string)
          }
        }
        n122 = call "FGV_HovaCAL_Interface_GetData.vi"("Aktion"=Aktion_FGV_HovaCAL_Interface_GetData."Limits", "Limits Cluster in"=w567) -> ()  [unwired: 5 in, 5 out]
      }
    }
  }
  "error out" <- w6
  "Aktion out" <- w5
  "connected?" <- w4
